vi "Detect Saccade Peak.vi"(4 "enum_direction":enum16{"Positive", "Negative"}(ring) caption="Impulse Direction", 5 "Impulse Data":refnum<data-value>, 6 "error in (no error)":errorcluster, 9 "Saccades in":T1[](array[typedef])) -> (0 "error out":errorcluster, 3 "Saccade out":T1[](array[typedef]))   [LabVIEW 2016]
uses:
  Type Definitions/Saccade Analyser Saccade Data.ctl
  Type Definitions/Saccade Analyser Impulse Data.ctl
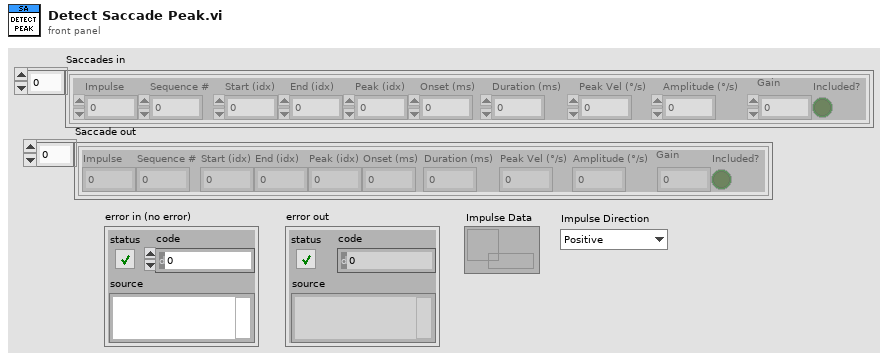
[diagram p1: front panel]
types:
  T1 = typedef "Saccade Analyser Saccade Data.ctl" = cluster{"Impulse":i32, "Sequence #":dbl, "Start (idx)":dbl, "End (idx)":dbl, "Peak (idx)":dbl, "Onset (ms)":dbl, "Duration (ms)":dbl, "Peak Vel (°/s)":dbl, "Amplitude (°/s)":dbl, "Gain":dbl, "Included?":bool}
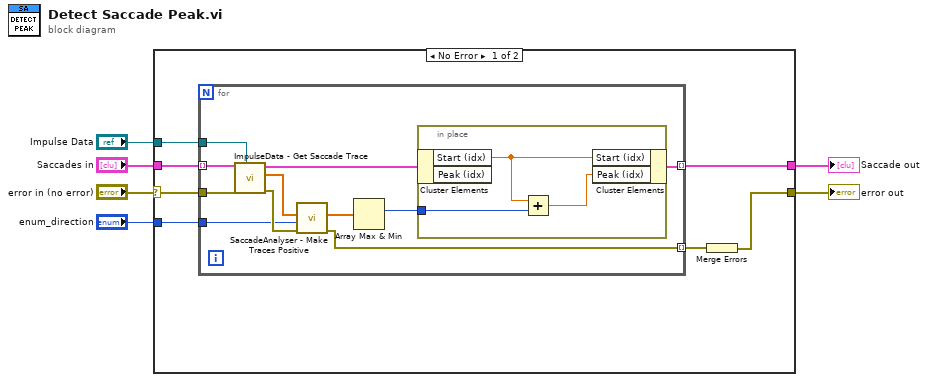
[diagram p0: block diagram]
diagram:
  n1 = case shown="No Error" "error in (no error)" {
    selector: "error in (no error)" -> [w11 w28]
    tunnel: "Saccades in" -> [w13 w29]
    tunnel: [w9 w29] -> w3
    tunnel: [w7 w28] -> w5
    tunnel: "Impulse Data" -> [w12 _]
    tunnel: "enum_direction" -> [w10 _]
    frame No Error {
      n2 = for {
        tunnel: w13 -> [w24] mode=indexing
        tunnel: w12 -> [w23]
        tunnel: w11 -> [w22]
        tunnel: w10 -> [w19]
        tunnel: [w14] -> w9 mode=indexing
        tunnel: [w16] -> w8 mode=indexing
        n3 = call "ImpulseData - Get Saccade Trace.vi"("Saccade in"=w24, "error in (no error)"=w22, "Impulse Data"=w23) -> ("Saccade out"=w15:T1, "Response Data"=w20:dbl[], "error out"=w21:errorcluster)  [unwired: 4 in, 1 out]
        n4 = call "SaccadeAnalyser - Make Traces Positive.vi"("error in (no error)"=w21, "enum_direction"=w19, "Response in"=w20) -> ("error out"=w16:errorcluster, "Response out"=w18:dbl[])  [unwired: 6 in, 1 out]
        n5 = Array Max & Min(array=w18) -> (max index (indices)=w17:i32)  [unwired: 3 out]
        n6 = in-place {
          in-place-border: w17 -> [w27]
          n7 = in-place-cluster #1(w15) -> ("Start (idx)"=w26:dbl)  [unwired: 1 out]
          n8 = Add(x=w26, y=w27) -> (x+y=w25:dbl)
          n9 = in-place-cluster #1("Start (idx)"=w26, "Peak (idx)"=w25) -> (w14:T1)
        }
      }
      n10 = Merge Errors(w8) -> (w7:errorcluster)
    }
    frame Error {
    }
  }
  "error out" <- w5
  "Saccade out" <- w3
